vi "Picohrdlerrorhandler.vi"(0 "Handle in":i16=16384, 1 "API function":string, 2 "Return":i16=-1, 3 "error in (no error)":errorcluster) -> (7 "Handle out":i16, 10 "error out":errorcluster)   [LabVIEW 2010]
uses:
  PicoHRDL.dll
panel:
  out "HRDL_SETTINGS":string
  out "HRDL_ERROR":string
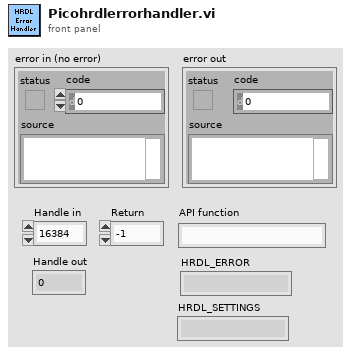
[diagram p1: front panel]
types:
  T1 = enum16{"HRDL_DRIVER_VERSION", "HRDL_USB_VERSION", "HRDL_HARDWARE_VERSION", "HRDL_VARIANT_INFO", "HRDL_BATCH_AND_SERIAL", "HRDL_CAL_DATE1", "HRDL_CAL_DATE2", "HRDL_ERROR", "HRDL_SETTINGS"}
  T2 = enum16{"Left Button", "Center Button", "Right Button", "Window Close"}
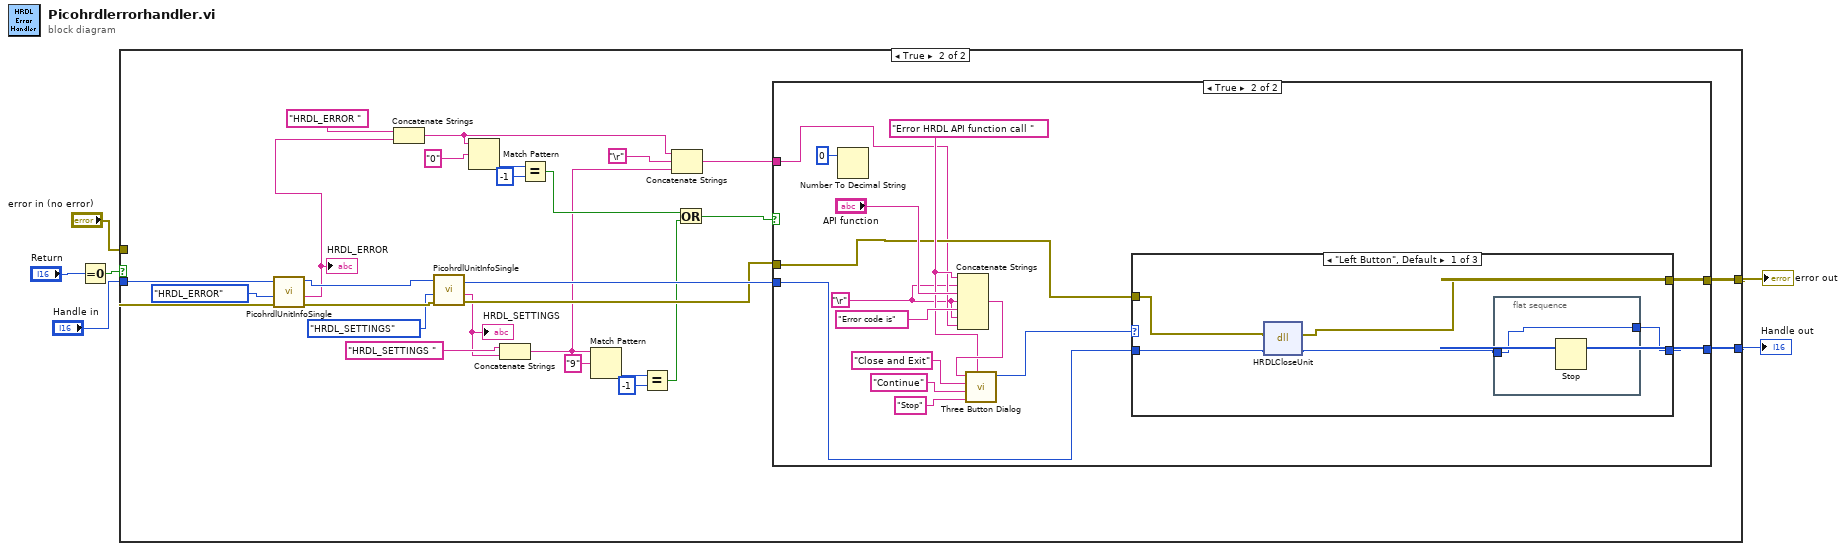
[diagram p0: block diagram]
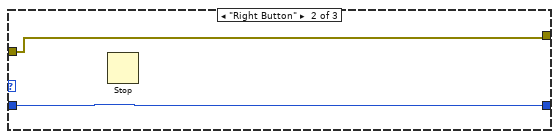
[diagram p4: hidden frame]
diagram:
  n1 = Equal To 0?(x="Return") -> (x = 0?=w4:bool)
  n2 = case shown="True" w4 {
    tunnel: "Handle in" -> [w8 w35]
    tunnel: [w8 w34] -> w3
    tunnel: "error in (no error)" -> [w7 w33]
    tunnel: [w7 w32] -> w1
    frame False {
    }
    frame True {
      n3 = call "PicohrdlUnitInfoSingle.vi"("error in (no error)"=w33, "info Enum"=T1."HRDL_ERROR", "Handle in"=w35) -> ("error out"=w27:errorcluster, "trimmed string"=w11:string, "handle out"=w31:i16)  [unwired: 5 in, 1 out]
      "HRDL_ERROR" <- w11
      n4 = Concatenate Strings("HRDL_ERROR " ("string"), w11) -> (w9:string)
      n5 = call "PicohrdlUnitInfoSingle.vi"("error in (no error)"=w27, "info Enum"=T1."HRDL_SETTINGS", "Handle in"=w31) -> ("error out"=w29:errorcluster, "trimmed string"=w13:string, "handle out"=w30:i16)  [unwired: 5 in, 1 out]
      "HRDL_SETTINGS" <- w13
      n6 = Match Pattern(string=w9, regular expression="0") -> (offset past match=w23:i32)  [unwired: 1 in, 3 out]
      n7 = Concatenate Strings("HRDL_SETTINGS " ("string"), w13) -> (w15:string)
      n8 = Equal?(x=w23, y=-1) -> (x = y?=w21:bool)
      n9 = Match Pattern(string=w15, regular expression="9") -> (offset past match=w20:i32)  [unwired: 1 in, 3 out]
      n10 = Equal?(x=w20, y=-1) -> (x = y?=w18:bool)
      n11 = Concatenate Strings(w9, "\r", w15) -> (w24:string)
      n12 = Or(x=w21, y=w18) -> (x .or. y?=w25:bool)
      n13 = case shown="True" w25 {
        tunnel: w30 -> [w37 w48]
        tunnel: [w37 w43] -> w34
        tunnel: w29 -> [w36 w42]
        tunnel: [w36 w41] -> w32
        tunnel: w24 -> [_ w39]
        frame False {
        }
        frame True {
          w38 = "\r"
          w44 = "Error HRDL API function call "
          n14 = Number To Decimal String(number=0) -> ()  [unwired: 1 in, 1 out]
          n15 = Concatenate Strings(w44, w38, "API function", w38, "Error code is" ("string"), w38, w39) -> (w47:string)
          n16 = call <vilib>:"Three Button Dialog.vi"("Window Title (\"\")"=w44, "Right Button Text (\"Cancel\")"="Stop" ("Right Button Text (\"Cancel\")"), "Center Button Text (\"No\")"="Continue" ("Center Button Text (\"No\")"), "Left Button Text (\"Yes\")"="Close and Exit" ("Left Button Text (\"Yes\")"), "message"=w47) -> ("Which Button?"=w49:T2)  [unwired: 6 in]
          n17 = case shown="\"Left Button\", Default" w49 {
            tunnel: w48 -> [w54 w60 w62]
            tunnel: [w57 w60 w62] -> w43
            tunnel: w42 -> [w56 w59 w61]
            tunnel: [w55 w59 w61] -> w41
            frame "Left Button", Default {
              n18 = dll-call lib="PicoHRDL.dll" fn="HRDLCloseUnit"(error in=w56, "handle"=w54) -> (error out=w55:errorcluster, "handle"=w53:i16)  [unwired: 3 in, 1 out]
              n19 = flat-sequence {
                tunnel: w53 -> [w58]
                tunnel: [w58] -> w57
                frame #0 {
                  n20 = Stop() -> ()  [unwired: 1 in]
                }
              }
            }
            frame "Right Button" {
              n21 = Stop() -> ()  [unwired: 1 in]
            }
            frame "Center Button" {
            }
          }
        }
      }
    }
  }
  "Handle out" <- w3
  "error out" <- w1
